vi "Add New Children.vi"(8 "error in (no error)":errorcluster, 9 "Folder Names":refnum<class "UTF-8 String.lvclass">[](array[class]), 10 "Parent Tag":refnum<class "UTF-8 String.lvclass">, 11 "Tree In":refnum<vi>) -> (0 "error out":errorcluster, 1 "Folder Names Dup":refnum<class "UTF-8 String.lvclass">[](array[class]), 2 "Parent Tag Dup":refnum<class "UTF-8 String.lvclass">, 3 "Tree Out":refnum<vi>)   [LabVIEW 2020, in "Tree Browser.lvlib"]
doc: "Adds new children under a parent node which exist on disk but not in the tree."
uses:
  Tree Browser.lvlib
  Types/UTF-8 String/UTF-8 String.lvclass
  Types/UTF-8 String/UTF-8 String.lvclass/UTF-8 String.ctl
  Unicode/Controls/Input String Encoding.ctl
  Types/UTF-8 Path/UTF-8 Path.lvclass/UTF-8 Path.ctl
  7b92c6cc-1de4-40f4-bc25-cd343e6c29a3.vi
  a1b79307-2118-473d-b28d-d385b1009f7d.vi
  7a5289d3-79ec-4b18-b602-64d5f2aa892c.vi
  Private/Conversion/String as Encoded String.vi
  Private/Conversion/Polymorphic VIs/String as Encoded String (UTF-8 String).vi
  Private/Conversion/Text as Encoded Path.vi
  Private/Conversion/Polymorphic VIs/Text as Encoded Path (UTF-8 String).vi
  Types/UTF-8 Path/Write Encoded UTF-8 Path.vi
  Private/Conversion/Path as Encoded Path.vi
  Private/Conversion/Polymorphic VIs/Path as Encoded Path (UTF-8 Path).vi
  Types/UTF-8 Path/Read Encoded UTF-8 Path.vi
  Private/Library/gu_strlen.vi
  Types/UTF-8 Path/UTF-8 Path.lvclass
  G-Unicode.lvlib
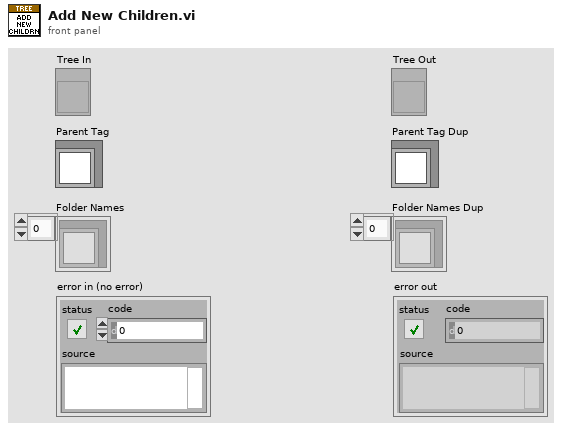
[diagram p1: front panel]
types:
  T1 = typedef "G-Unicode.lvlib/Input String Encoding.ctl" = enum16{"ANSI", "UTF-8", "UTF-16LE", "UTF-16BE", "Auto"}
  T2 = typedef "G-Unicode.lvlib/Encoded UTF-8 String.ctl" = string
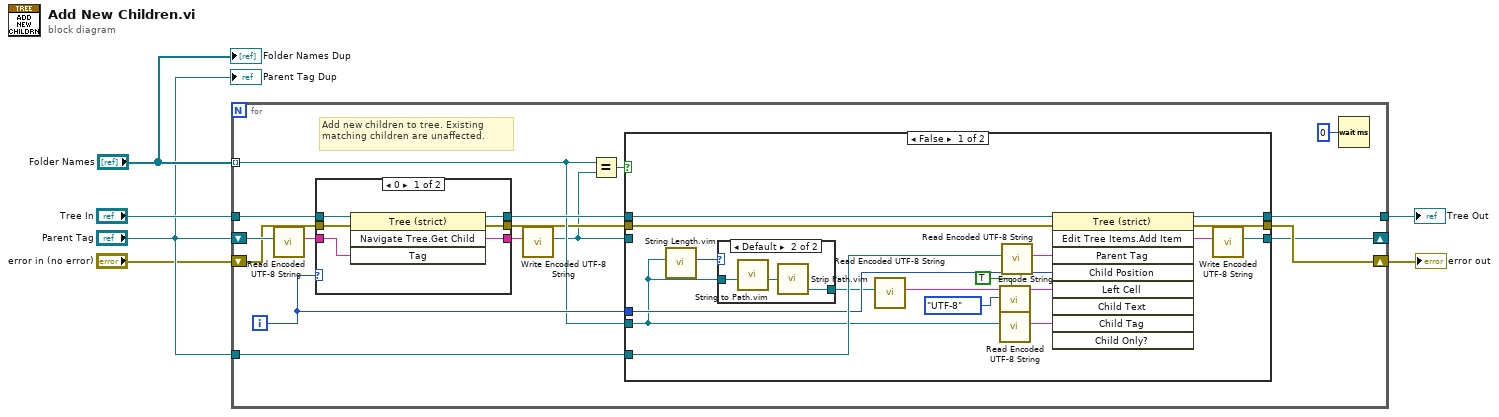
[diagram p0: block diagram]
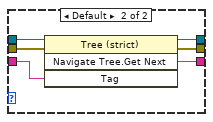
[diagram p4: hidden frame]
diagram:
  n1 = for {
    tunnel: "Tree In" -> [w22]
    shift-right: [w11] -> _
    shift-left: "Parent Tag" -> [w21]
    tunnel: "Folder Names" -> [w17] mode=indexing
    tunnel: "Parent Tag" -> [w20]
    tunnel: [w15] -> w4
    shift-right: [w12] -> w1
    shift-left: "error in (no error)" -> [w14]
    i -> [w18]
    # "Add new children to tree. Existing matching children are unaffected."
    n2 = call "Read Encoded UTF-8 String.vi"("UTF-8 String"=w21) -> ("Encoded UTF-8 String"=w8:T2)  [unwired: 10 in]
    n3 = case shown="0" w18 {
      tunnel: w22 -> [w52 w58]
      tunnel: w8 -> [w51 w57]
      tunnel: [w50 w56] -> w10
      tunnel: [w49 w55] -> w19
      tunnel: w14 -> [w48 w54]
      tunnel: [w47 w53] -> w13
      frame 0 {
        n4 = invoke class="Tree (strict)" method="Navigate Tree.Get Child"(reference=w52, error in=w48, "Tag"=w51) -> (reference out=w49:refnum<vi>, error out=w47:errorcluster, "Navigate Tree:Get Child"=w50:string)  [unwired: 1 in, 1 out]
      }
      frame Default {
        n5 = invoke class="Tree (strict)" method="Navigate Tree.Get Next"(reference=w58, error in=w54, "Tag"=w57) -> (reference out=w55:refnum<vi>, error out=w53:errorcluster, "Navigate Tree:Get Next Item"=w56:string)  [unwired: 1 in, 1 out]
      }
    }
    n6 = call "Write Encoded UTF-8 String.vi"("Encoded UTF-8 String"=w10) -> ("UTF-8 String"=w7:refnum<class "UTF-8 String.lvclass">)  [unwired: 10 in]
    n7 = Equal?(x=w17, y=w7) -> (x = y?=w16:bool)
    n8 = case shown="False" w16 {
      tunnel: w20 -> [w39 _]
      tunnel: w19 -> [w38 w46]
      tunnel: w18 -> [w37 _]
      tunnel: w17 -> [w31 _]
      tunnel: [w36 w46] -> w15
      tunnel: w13 -> [w35 w45]
      tunnel: [w34 w45] -> w12
      tunnel: [w27 w44] -> w11
      tunnel: w7 -> [_ w44]
      frame False {
        n9 = call "String Length.vim"("String"=w31) -> ("Length"=w30:i32)  [unwired: 9 in, 1 out]
        n10 = case shown="Default" w30 {
          tunnel: w31 -> [w40 w42]
          tunnel: [w40 w41] -> w33
          frame 3 {
          }
          frame Default {
            n11 = call "String to Path.vim"("String"=w42) -> ("Path"=w43:refnum<class "UTF-8 Path.lvclass">)  [unwired: 9 in, 1 out]
            n12 = call "Strip Path.vim"("Path"=w43) -> ("Name"=w41:refnum<class "UTF-8 String.lvclass">)  [unwired: 6 in, 2 out]
          }
        }
        n13 = call "Read Encoded UTF-8 String.vi"("UTF-8 String"=w33) -> ("Encoded UTF-8 String"=w26:T2)  [unwired: 10 in]
        n14 = call "Encode String.vi"("Prepend BOM (F)"=TRUE, "Input Encoding (ANSI)"=Input_String_Encoding."UTF-8", "String in"=w26) -> ("String out"=w25:string)  [unwired: 7 in, 1 out]
        n15 = call "Read Encoded UTF-8 String.vi"("UTF-8 String"=w31) -> ("Encoded UTF-8 String"=w28:T2)  [unwired: 10 in]
        n16 = call "Read Encoded UTF-8 String.vi"("UTF-8 String"=w39) -> ("Encoded UTF-8 String"=w29:T2)  [unwired: 10 in]
        n17 = invoke class="Tree (strict)" method="Edit Tree Items.Add Item"(reference=w38, error in=w35, "Parent Tag"=w29, "Child Position"=w37, "Left Cell"=w25, "Child Tag"=w28) -> (reference out=w36:refnum<vi>, error out=w34:errorcluster, "Edit Tree Items:Add Item"=w32:string)  [unwired: 3 in, 6 out]
        n18 = call "Write Encoded UTF-8 String.vi"("Encoded UTF-8 String"=w32) -> ("UTF-8 String"=w27:refnum<class "UTF-8 String.lvclass">)  [unwired: 10 in]
      }
      frame True {
      }
    }
    n19 = Wait (ms)(milliseconds to wait=u32 0) -> ()  [unwired: 1 out]
  }
  "Tree Out" <- w4
  "error out" <- w1
  "Parent Tag Dup" <- "Parent Tag"
  "Folder Names Dup" <- "Folder Names"
